vi "Read 1553 Channel Handles.vi"(8 "error in":errorcluster, 11 "Execution Unit in":refnum<class "Execution Unit.lvclass">) -> (0 "error out":errorcluster, 2 "1553 channel handles":T1[](array[typedef]) {"terminal status channels" format="%.0x"; "messages"."Rx status handles" format="%.0x"; "messages"."Tx status handles" format="%.0x"; "messages"."timestamps" format="%.0x"; "messages"."parameters"."RxBC channel handle" format="%.0x"; "messages"."parameters"."RxRT channel handle" format="%.0x"; "messages"."parameters"."Tx channel handle" format="%.0x"}, 3 "Execution Unit out":refnum<class "Execution Unit.lvclass">)   [LabVIEW 2020, in "AIM MIL-STD-1553 Engine.lvlib" / "Implementation.lvlib" / "Execution Unit.lvclass"]
uses:
  Execution Unit.lvclass
  <vilib>/NI VeriStand/Custom Device API/Custom Device Item Ref.ctl
  <vilib>/NI VeriStand/Custom Device API/Custom Device API.lvlib
  Parameter Handles.ctl
  Message Handles.ctl
  Shared/1553 Channel Handles.ctl
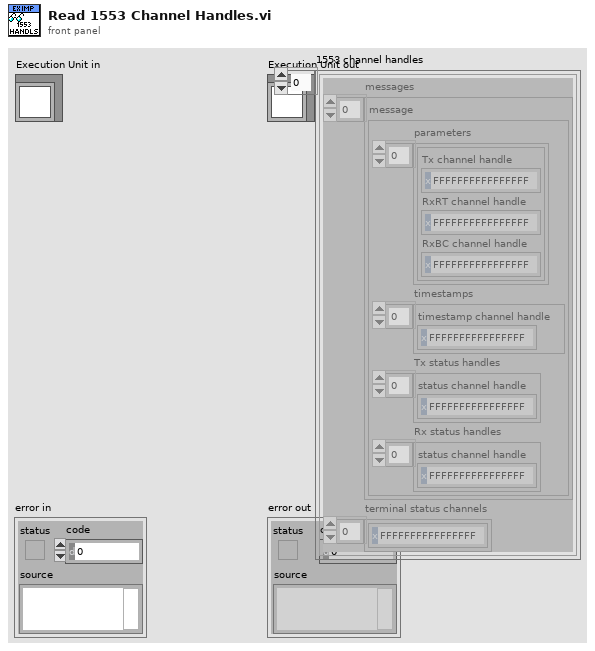
[diagram p1: front panel]
types:
  T1 = typedef "1553 Channel Handles.ctl" = cluster{"messages":T2[], "terminal status channels":T4[]}
  T2 = typedef "AIM MIL-STD-1553 Engine.lvlib/Implementation.lvlib/Execution Unit.lvclass/Message Handles.ctl" = cluster{"parameters":T3[], "timestamps":T4[], "Tx status handles":T4[], "Rx status handles":T4[]}
  T3 = typedef "AIM MIL-STD-1553 Engine.lvlib/Implementation.lvlib/Execution Unit.lvclass/Parameter Handles.ctl" = cluster{"Tx channel handle":T4, "RxRT channel handle":T4, "RxBC channel handle":T4}
  T4 = typedef "Custom Device API.lvlib/Custom Device Item Ref.ctl" = u64
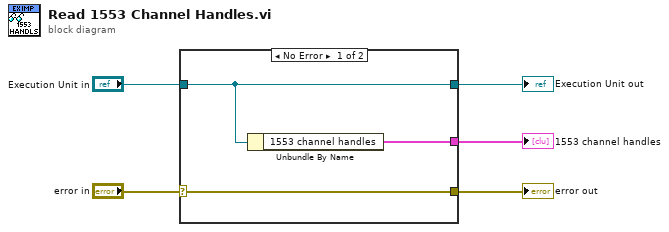
[diagram p0: block diagram]
diagram:
  n1 = case shown="No Error" "error in" {
    selector: "error in" -> [w8 w9]
    tunnel: [w8 w9] -> w4
    tunnel: [w7 w10] -> w2
    tunnel: "Execution Unit in" -> [w7 w10]
    tunnel: [w6 _] -> w1
    frame No Error {
      n2 = Unbundle By Name(w7) -> ("1553 channel handles"=w6:T1[])
    }
    frame Error {
    }
  }
  "error out" <- w4
  "Execution Unit out" <- w2
  "1553 channel handles" <- w1
